vi "Boxplot - Create Box Array.vi"(5 "delta x":dbl=2.5 format="%#.6g", 7 "x":dbl=1.0 format="%#.6g", 9 "Lower quartile (LQ)":dbl=1.5 format="%#.6g", 10 "Median":dbl=3.0 format="%#.6g", 11 "Upper quartile (UQ)":dbl=4.5 format="%#.6g") -> (3 "XY Graph":cluster{dbl[], dbl[]}(graph))   [LabVIEW 2023]
doc: "Computes the array data for graphing the boxplot."
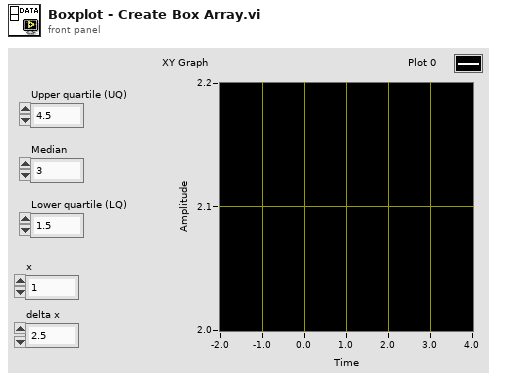
[diagram p1: front panel]
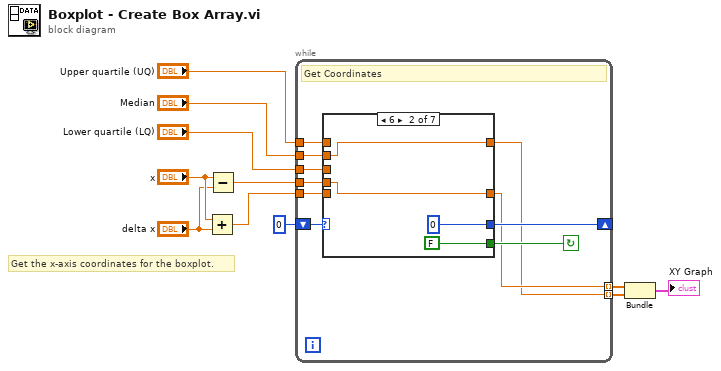
[diagram p0: block diagram]
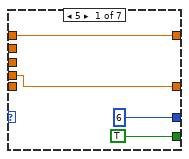
[diagram p2: hidden frame]
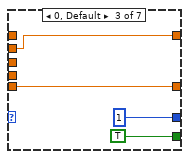
[diagram p3: hidden frame]
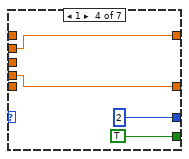
[diagram p4: hidden frame]
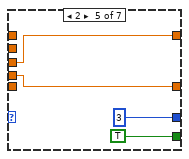
[diagram p5: hidden frame]
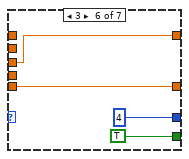
[diagram p6: hidden frame]
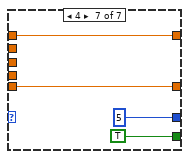
[diagram p7: hidden frame]
diagram:
  # "Get the x-axis coordinates for the boxplot."
  n1 = Add(x="x", y="delta x") -> (x+y=w5:dbl)
  n2 = Subtract(x="x", y="delta x") -> (x-y=w6:dbl)
  n3 = while {
    shift-right: [w21] -> _
    shift-left: 0 -> [w20]
    tunnel: "Upper quartile (UQ)" -> [w18]
    tunnel: "Median" -> [w17]
    tunnel: "Lower quartile (LQ)" -> [w16]
    tunnel: w6 -> [w15]
    tunnel: w5 -> [w14]
    tunnel: [w13] -> w2 mode=indexing
    tunnel: [w12] -> w1 mode=indexing
    stop <- w19 continue-if-true
    # "Get Coordinates"
    n4 = case shown="6" w20 {
      tunnel: [6 0 1 2 3 4 5] -> w21
      tunnel: [TRUE FALSE TRUE TRUE TRUE TRUE TRUE] -> w19
      tunnel: w18 -> [w23 _ _ _ _ _ w46]
      tunnel: w17 -> [_ w27 w30 w34 _ _ _]
      tunnel: w16 -> [_ _ _ _ w38 w42 _]
      tunnel: w15 -> [w24 w28 _ w35 w39 _ _]
      tunnel: w14 -> [_ _ w31 _ _ w43 w47]
      tunnel: [w24 w28 w31 w35 w39 w43 w47] -> w13
      tunnel: [w23 w27 w30 w34 w38 w42 w46] -> w12
      frame 5 {
      }
      frame 6 {
      }
      frame 0, Default {
      }
      frame 1 {
      }
      frame 2 {
      }
      frame 3 {
      }
      frame 4 {
      }
    }
  }
  n5 = Bundle(w2, w1) -> (→"XY Graph":cluster{dbl[], dbl[]})  [unwired: 1 in]
